vi "Write x (800).vi"(8 "error in (no error)":errorcluster, 10 "x (800)":i16=800, 11 "cosmetic changes in":refnum<class "cosmetic changes.lvclass">) -> (0 "error out":errorcluster, 3 "cosmetic changes out":refnum<class "cosmetic changes.lvclass">)   [LabVIEW 2013, in "cosmetic changes.lvclass"]
uses:
  cosmetic changes.lvclass
  cosmetic changes.lvclass/cosmetic changes.ctl
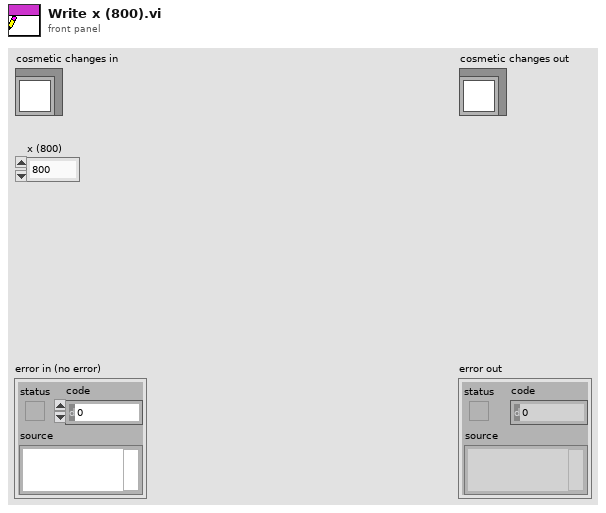
[diagram p1: front panel]
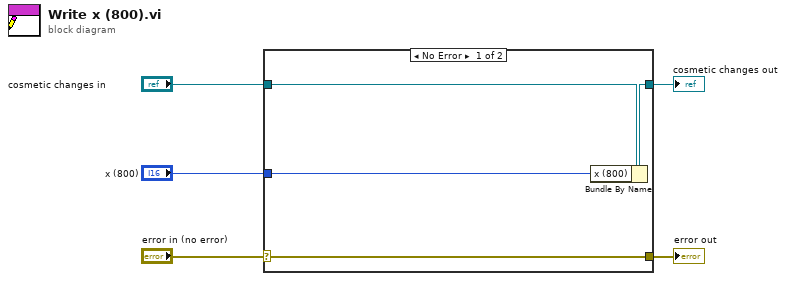
[diagram p0: block diagram]
diagram:
  n1 = case shown="No Error" "error in (no error)" {
    selector: "error in (no error)" -> [w9 w10]
    tunnel: [w9 w10] -> w4
    tunnel: [w7 w11] -> w2
    tunnel: "cosmetic changes in" -> [w8 w11]
    tunnel: "x (800)" -> [w6 _]
    frame No Error {
      n2 = Bundle By Name(cluster=w8, "x (800)"=w6) -> (w7:refnum<class "cosmetic changes.lvclass">)
    }
    frame Error {
    }
  }
  "error out" <- w4
  "cosmetic changes out" <- w2
